vi "cluster.vi"() -> ()   [LabVIEW 2013]
panel:
  out "success2":bool
  in  "Cluster 2":T1
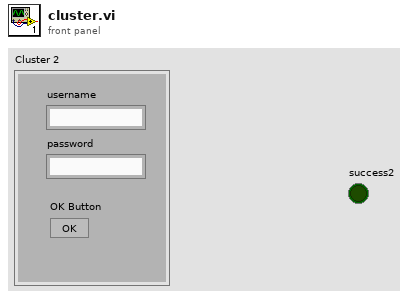
[diagram p1: front panel]
types:
  T1 = cluster{"username":string, "password":string, "OK Button":bool}
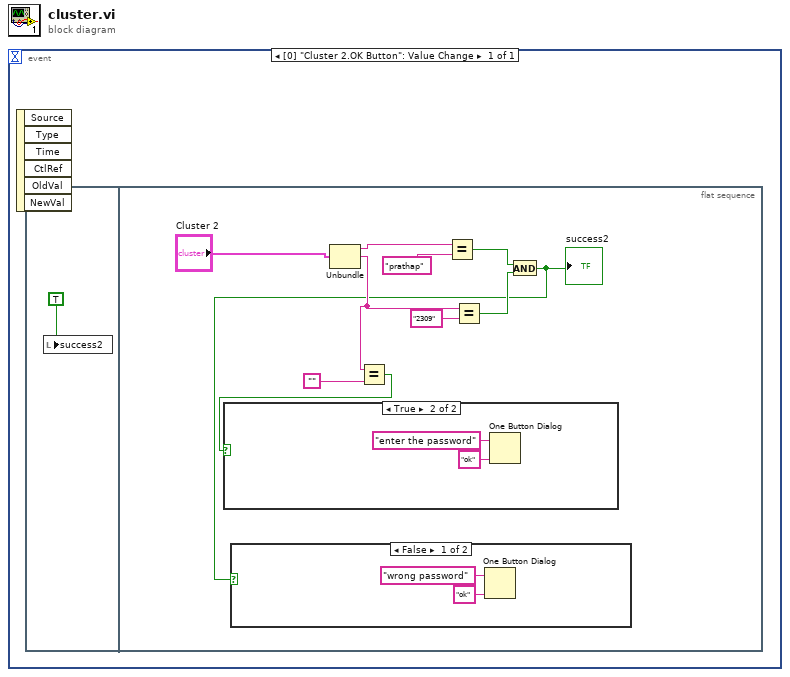
[diagram p0: block diagram]
diagram:
  n1 = event shown="[0] \"Cluster 2.OK Button\": Value Change" {
    selector: _ -> [_]
    dyn-events: _ -> [_]
    timeout: _ -> [_]
    event "Cluster 2.OK Button": Value Change {
      n2 = event-data() -> ()  [unwired: 1 in, 6 out]
      n3 = flat-sequence {
        frame #0 {
          n4 = local write "success2"(TRUE) -> ()
        }
        frame #1 {
          n5 = Unbundle("Cluster 2") -> ("username"=w10:string, "password"=w8:string)  [unwired: 1 out]
          n6 = Equal?(x=w8, y="") -> (x = y?=w3:bool)
          n7 = case shown="True" w3 {
            frame False {
            }
            frame True {
              n8 = One Button Dialog(message="enter the password", button name ("OK")="ok") -> ()  [unwired: 1 out]
            }
          }
          n9 = Equal?(x=w10, y="prathap") -> (x = y?=w6:bool)
          n10 = Equal?(x=w8, y="2309") -> (x = y?=w5:bool)
          n11 = And(x=w6, y=w5) -> (x .and. y?=w2:bool)
          "success2" <- w2
          n12 = case shown="False" w2 {
            frame False {
              n13 = One Button Dialog(message="wrong password", button name ("OK")="ok") -> ()  [unwired: 1 out]
            }
            frame True {
            }
          }
        }
      }
    }
  }
